vi "find device.vi"(10 "Device Description":string, 11 "List of devices":T1 {"List of locations"."Position"."Position Y" format="%#.3f"; "List of locations"."Position"."Position X" format="%#.3f"}) -> (1 "Index of device":i32, 2 "Found?":bool, 3 "Defualt Device":T2 {"List of locations"."Position"."Position Y" format="%#.3f"; "List of locations"."Position"."Position X" format="%#.3f"})   [LabVIEW 2017]
uses:
  device.ctl
  location.ctl
  device_list.ctl
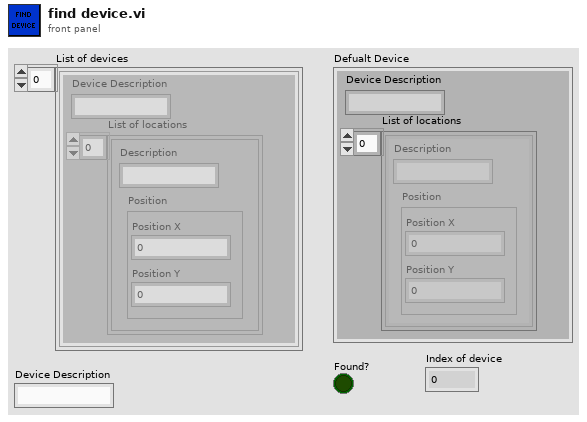
[diagram p1: front panel]
types:
  T1 = typedef "device_list.ctl" = T2[]
  T2 = typedef "device.ctl" = cluster{"List of locations":T3[], "Device Description":string}
  T3 = typedef "location.ctl" = cluster{"Description":string, "Position":cluster{"Position X":dbl, "Position Y":dbl}}
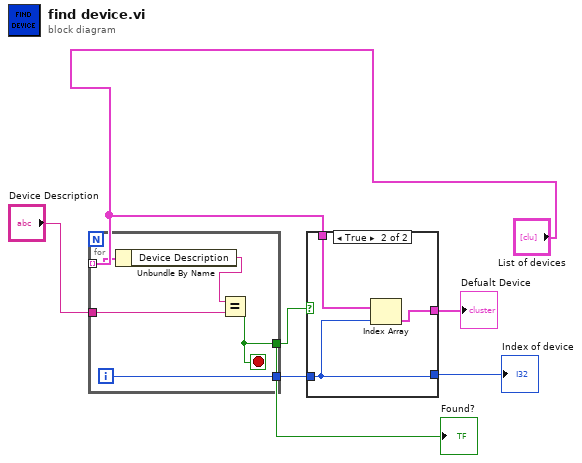
[diagram p0: block diagram]
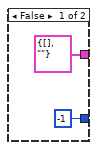
[diagram p2: hidden frame]
diagram:
  n1 = for {
    tunnel: "List of devices" -> [w11] mode=indexing
    tunnel: "Device Description" -> [w9]
    tunnel: [w8] -> w3
    tunnel: [w7] -> w4
    i -> [w7]
    stop <- w8 stop-if-true
    n2 = Unbundle By Name(w11) -> ("Device Description"=w10:string)
    n3 = Equal?(x=w10, y=w9) -> (x = y?=w8:bool)
  }
  "Found?" <- w3
  n4 = case shown="True" w3 {
    tunnel: w4 -> [_ w14]
    tunnel: "List of devices" -> [_ w16]
    tunnel: [T2 {"List of locations"=[], "Device Description"=""} ("Defualt Device") w15] -> w6
    tunnel: [-1 w14] -> w1
    frame False {
    }
    frame True {
      n5 = Index Array(array=w16, index=w14) -> (element=w15:T2)
    }
  }
  "Defualt Device" <- w6
  "Index of device" <- w1
